vi "VerifyArmStatus.vi"() -> (11 "Is Arm Up?":bool)   [LabVIEW 2016, in "LEGO-PMR.lvrbt"]
uses:
  LEGO-PMR.lvrbt
  <vilib>/NXT/Block Support/NXT_ButtonSelector.ctl
  <vilib>/NXT/Dual Mode Library/Display/drawText.vi
  <vilib>/NXT/Dual Mode Library/Sensors/readNXTButton.vi
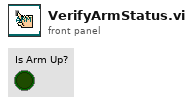
[diagram p1: front panel]
types:
  T1 = typedef "NXT_ButtonSelector.ctl" = u16
  T2 = typedef "LVHSConnector.ctl" = refnum<class "BrickReference.lvclass">
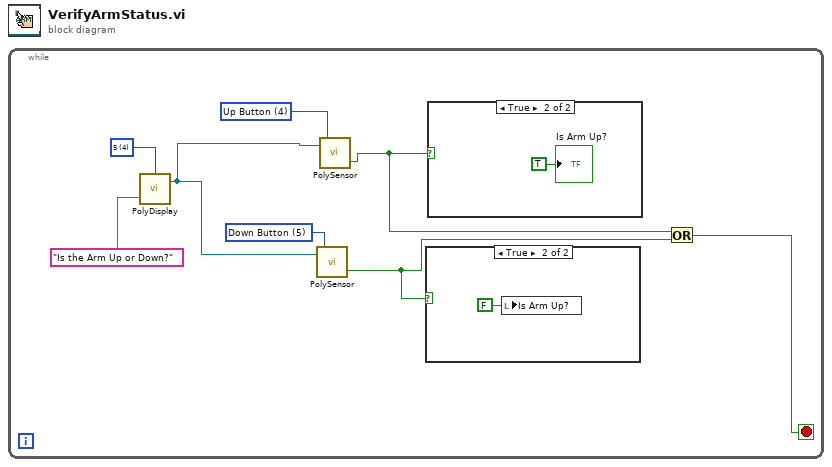
[diagram p0: block diagram]
diagram:
  n1 = while {
    stop <- w1 stop-if-true
    w6 = T1 5 items=["Enter button"=3, "Left button"=2, "Right button"=1, "Up Button"=4, "Down Button"=5] ("Button (Enter button)")
    w5 = T1 4 items=["Enter button"=3, "Left button"=2, "Right button"=1, "Up Button"=4, "Down Button"=5] ("Button (Enter button)")
    w8 = i16 4 items=["1", "2", "3", "4", "5", "6", "7", "8", "9", "10", "11", "12"] ("Line")
    n2 = call-poly <vilib>:"PolyDisplay.vi"("Text"="Is the Arm Up or Down?", "Line"=w8) -> ("NXT/EV3"=w4:T2)  [unwired: 2 in]
    n3 = call-poly <vilib>:"PolySensor.vi"("Button (Enter button)"=w6, "NXT/EV3"=w4) -> ("Yes/No"=w2:bool)  [unwired: 1 in, 1 out]
    n4 = call-poly <vilib>:"PolySensor.vi"("Button (Enter button)"=w5, "NXT/EV3"=w4) -> ("Yes/No"=w3:bool)  [unwired: 1 in, 1 out]
    n5 = case shown="True" w2 {
      frame False {
      }
      frame True {
        n6 = local write "Is Arm Up?"(FALSE ("Is Arm Up?")) -> ()
      }
    }
    n7 = case shown="True" w3 {
      frame False {
      }
      frame True {
        "Is Arm Up?" <- TRUE ("Is Arm Up?")
      }
    }
    n8 = Or(x=w3, y=w2) -> (x .or. y?=w1:bool)
  }
